vi "Data.vi"(11 "Override Error Msg in":refnum<class "Override Error Msg.lvclass">) -> (2 "Error":errorcluster)   [LabVIEW 2021, in "Override Error.lvlib" / "Override Error Msg.lvclass"]
uses:
  Override Error Msg.lvclass
  Override Error Msg.lvclass/Override Error Msg.ctl
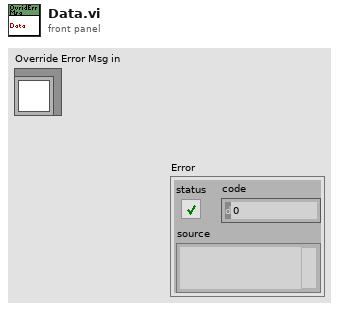
[diagram p1: front panel]
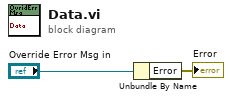
[diagram p0: block diagram]
diagram:
  n1 = Unbundle By Name("Override Error Msg in") -> ("Error"=→"Error":errorcluster)
